vi "Get Files.vi"() -> ()   [LabVIEW 2014]
panel:
  out "folder names":string[](array[string])
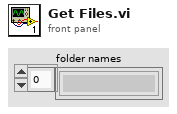
[diagram p1: front panel]
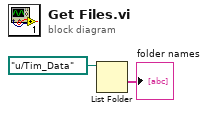
[diagram p0: block diagram]
diagram:
  n1 = List Folder(path=path "u:/Tim_Data") -> (folder names=→"folder names":string[])  [unwired: 3 in, 3 out]
